vi "Recovery Format SN.vi"(8 "error in (no error)":errorcluster caption="entrée d'erreur (pas d'erreur)", 11 "Firebase Benches en entrée":refnum<class "Firebase Recovery_SN.lvclass">) -> (0 "error out":errorcluster caption="sortie d'erreur", 3 "Firebase Benches en sortie":refnum<class "Firebase Recovery_SN.lvclass">)   [LabVIEW 2020, in "Library Instrument & Equipement.lvlib" / "Library FireBase.lvlib" / "Firebase Recovery_SN.lvclass"]
doc: "Returns data according to Value_To_Find on Collection_to_find Use Nb_To_Read to determine the number to read\nPlease initialise the following values before use the VI\n - Name BDD\n - Value to find\n - API Key\n - Field Filter\n - Field Order\n - Collection_to_find\n\nIf there is no Field order -> Field Order=Field Filter"
uses:
  Firebase Recovery_SN.lvclass
  C:/Users/ngarcin/OneDrive - Altyor/Standard TB/Class/Firebase/Source/Firebase Driver/Firebase Driver.lvclass
  Firebase Recovery_SN.lvclass/Firebase Recovery_SN.ctl
  JSON API/JSON Value/Set from JSON string.vi
  JSON API/JSON Value/JSON Value.lvclass
  JSON API/Variant JSON/Variant JSON.lvlib
  JSON API/Get Polymorphic/JSON GetSet.lvlib
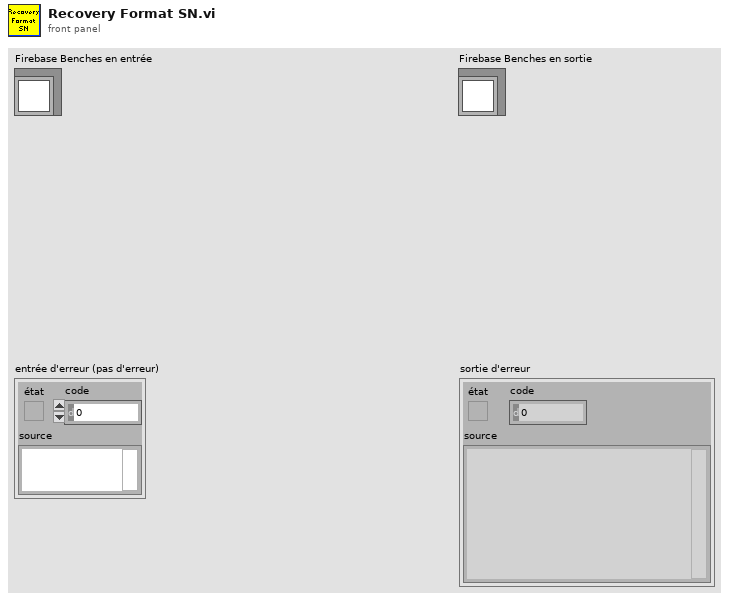
[diagram p1: front panel]
types:
  T1 = cluster{"name":string, "fields":cluster{"Format":cluster{"stringValue":string}}}[]
  T2 = cluster{"name":string, "fields":cluster{"Format":cluster{"stringValue":string}}}
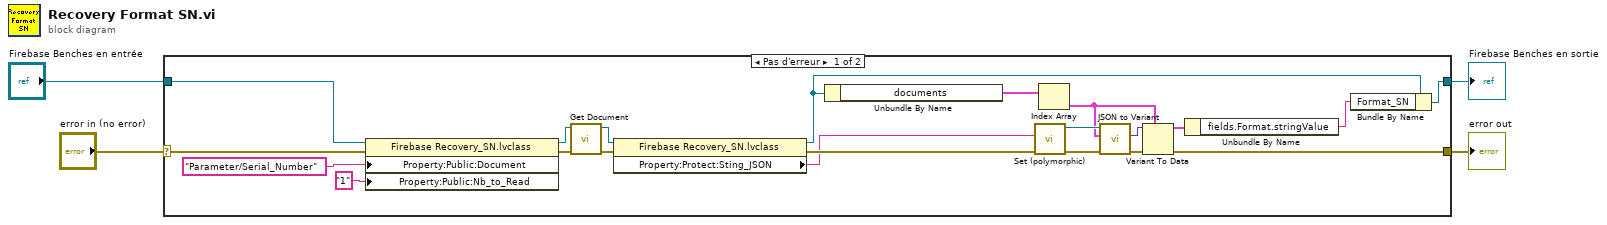
[diagram p0: block diagram]
diagram:
  n1 = case shown="Pas d'erreur" "error in (no error)" {
    selector: "error in (no error)" -> [w24 w27]
    tunnel: "Firebase Benches en entrée" -> [w25 w26]
    tunnel: [w22 w27] -> w3
    tunnel: [w23 w26] -> w2
    frame No Error {
      n2 = property class="Firebase Recovery_SN.lvclass"(reference=w25, error in=w24, "Property:Public:Document"="Parameter/Serial_Number" ("Collection_to_find"), "Property:Public:Nb_to_Read"="1" ("Nb_to_Read")) -> (reference out=w19:refnum<class "Firebase Recovery_SN.lvclass">, error out=w20:errorcluster)
      n3 = call-dynamic "Get Document.vi"("error in (no error)"=w20, "Firebase (Default) en entrée"=w19) -> ("error out"=w11:errorcluster, "Firebase (Default) en sortie"=w10:refnum<class "Firebase Recovery_SN.lvclass">)  [unwired: 8 in]
      n4 = property class="Firebase Recovery_SN.lvclass"(reference=w10, error in=w11) -> (reference out=w9:refnum<class "Firebase Recovery_SN.lvclass">, error out=w16:errorcluster, "Property:Protect:Sting_JSON"=w15:string)
      n5 = Unbundle By Name(w9) -> ("documents"=w7:T1)
      n6 = call-poly "Set (polymorphic).vi"("error in (no error)"=w16, "JSON stream"=w15) -> ("error out"=w14:errorcluster, "JSON Value out"=w12:refnum<class "JSON Value.lvclass">)  [unwired: 7 in, 1 out]
      n7 = Index Array(array=w7) -> (element=w5:T2)  [unwired: 1 in]
      n8 = call "JSON to Variant.vi"("error in (no error)"=w14, "Variant (Data Type)"=w5, "JSON Value"=w12) -> ("error out"=w13:errorcluster, "Variant out"=w17:variant)  [unwired: 7 in]
      n9 = Variant To Data(error in=w13, type=w5, Variant=w17) -> (data=w6:T2, error out=w22:errorcluster)
      n10 = Unbundle By Name(w6) -> ("fields.Format.stringValue"=w8:string)
      n11 = Bundle By Name(cluster=w9, "Format_SN"=w8) -> (w23:refnum<class "Firebase Recovery_SN.lvclass">)
    }
    frame Error {
    }
  }
  "error out" <- w3
  "Firebase Benches en sortie" <- w2
